vi "获取起始位置.vi"(8 "error in (no error)":errorcluster caption="错误输入（无错误）", 10 "起始坐标":cluster{"Horizontal":i32, "Vertical":i32}, 11 "程序响应 输入":refnum<class "程序响应.lvclass">) -> (0 "error out":errorcluster caption="错误输出", 3 "程序响应 输出":refnum<class "程序响应.lvclass">)   [LabVIEW 2020, in "程序响应.lvlib" / "程序响应.lvclass"]
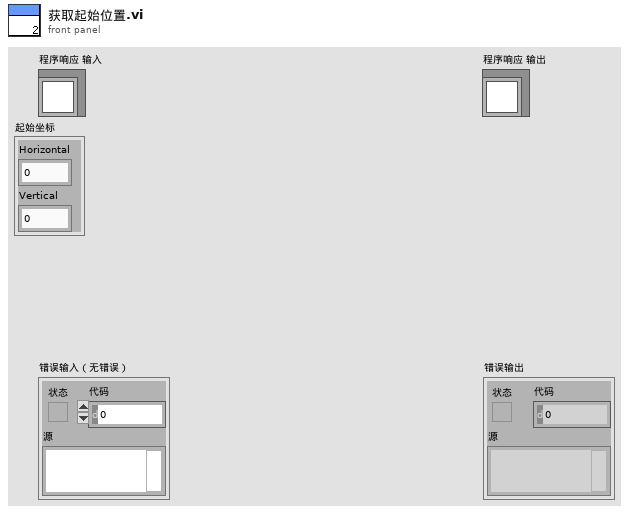
[diagram p1: front panel]
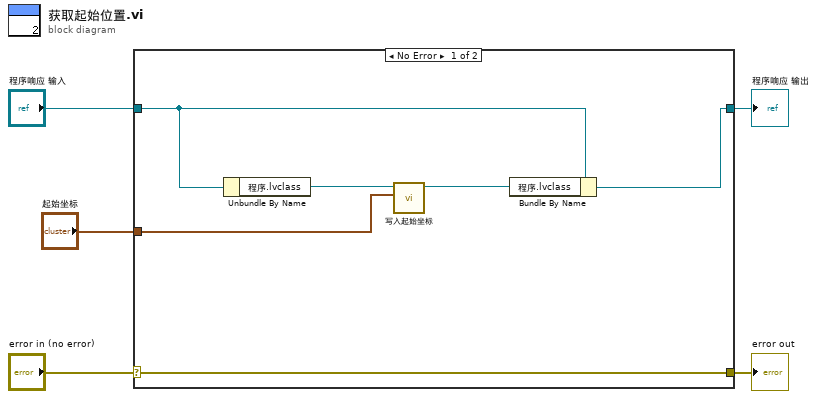
[diagram p0: block diagram]
diagram:
  n1 = case shown="No Error" "error in (no error)" {
    selector: "error in (no error)" -> [w11 w13]
    tunnel: [w11 w13] -> w4
    tunnel: [w7 w12] -> w2
    tunnel: "程序响应 输入" -> [w9 w12]
    tunnel: "起始坐标" -> [w6 _]
    frame No Error {
      n2 = Unbundle By Name(w9) -> ("程序.lvclass"=w10:refnum<class "程序.lvclass">)
      n3 = call-dynamic "写入起始坐标.vi"("起始坐标"=w6, "程序输入"=w10) -> ("程序输出"=w8:refnum<class "程序.lvclass">)  [unwired: 8 in, 1 out]
      n4 = Bundle By Name(cluster=w9, "程序.lvclass"=w8) -> (w7:refnum<class "程序响应.lvclass">)
    }
    frame Error {
    }
  }
  "error out" <- w4
  "程序响应 输出" <- w2
